vi "FTW-CodeGen-JSON-Bounds.vi"(0 "State In":T1, 5 "XRef":refnum<vi>) -> (4 "Bounds":cluster{"Width":i32, "Height":i32})   [LabVIEW 2012, in "FTW-JSON-Deserialize.xnode"]
uses:
  src/JSON/FTW-JSON-Deserialize.xnode
  FTW-CodeGen-JSON-State.ctl
panel:
  # "Inputs"
  # "Outputs"
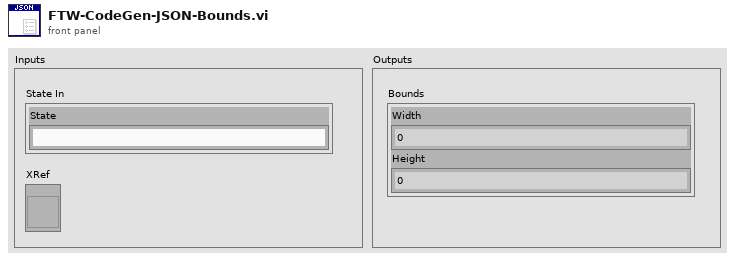
[diagram p1: front panel]
types:
  T1 = typedef "FTW-JSON-Deserialize.xnode/FTW-CodeGen-JSON-State.ctl" = cluster{"State":string}
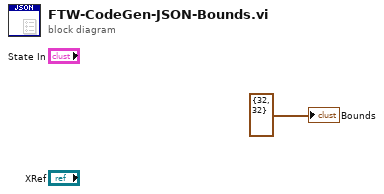
[diagram p0: block diagram]
diagram:
  "Bounds" <- cluster{"Width":i32, "Height":i32} {"Width"=32, "Height"=32} ("Bounds")
